vi "UDP Streamer.vi"() -> ()   [LabVIEW 2017]
panel:
  out "#Clients":u32
  in  "Stop":bool
  in  "Delay":i32(knob)=19 caption="Send Packet Every (ms)" min=1 scale=1.0..200.0
  in  "Size":i32(knob)=17515 caption="UDP Data Packet Size (bytes)" min=1 scale=0.0..100000.0 scale format="%#_6p"
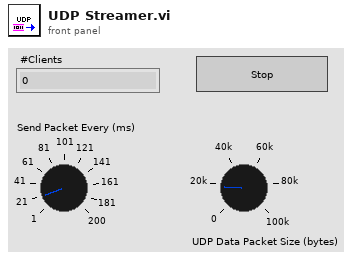
[diagram p1: front panel]
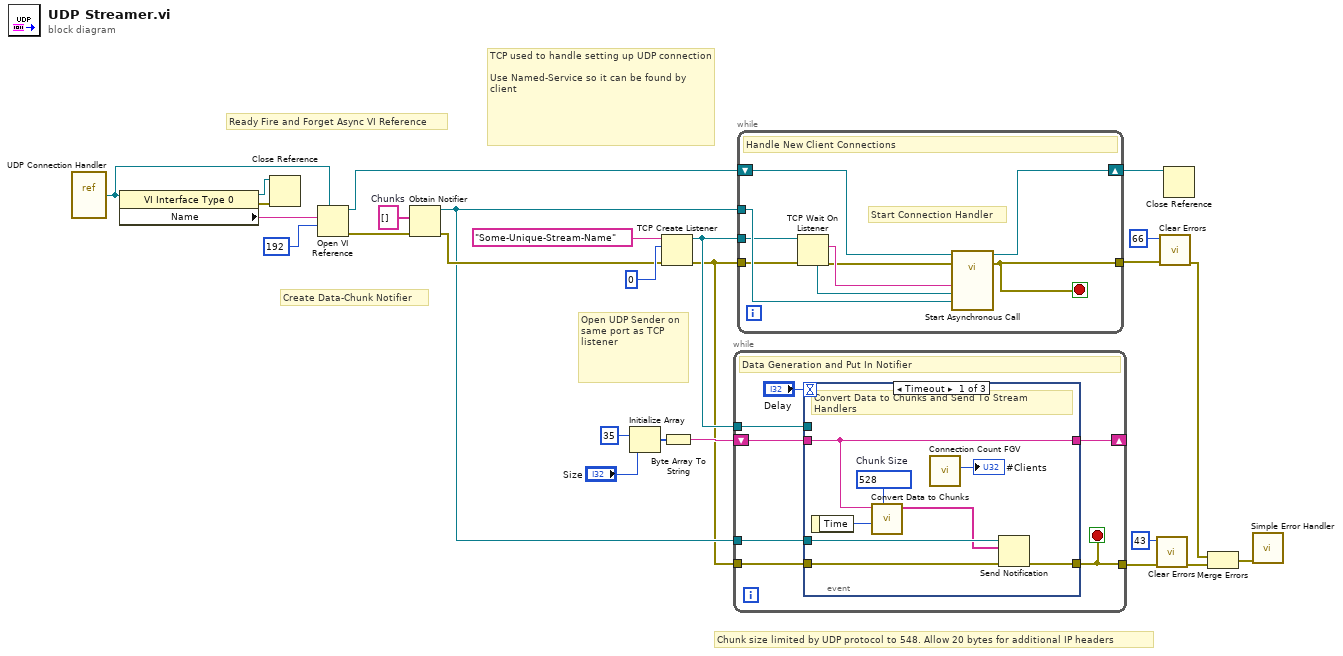
[diagram p0: block diagram]
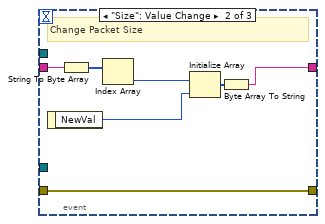
[diagram p2: hidden frame]
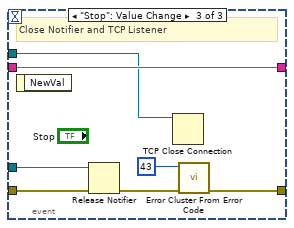
[diagram p3: hidden frame]
diagram:
  w14 = string[] []  # Chunks
  # "Chunk size limited by UDP protocol to 548. Allow 20 bytes for additional IP headers"
  # "Open UDP Sender on same port as TCP listener"
  # "TCP used to handle setting up UDP connection\n\nUse Named-Service so it can be found by client"
  # "Create Data-Chunk Notifier"
  # "Ready Fire and Forget Async VI Reference"
  n1 = vi-ref "UDP Connection Handler.vi"() -> (w10:refnum<vi>)
  n2 = property class="VI Interface Type 0"(reference=w10) -> (reference out=w8:refnum<vi>, error out=w9:errorcluster, "Name"=w11:string)  [unwired: 1 in]
  n3 = Close Reference(reference=w8, error in (no error)=w9) -> ()  [unwired: 1 out]
  n4 = Open VI Reference(type specifier VI Refnum (for type only)=w10, vi path=w11, options=192) -> (vi reference=w5:refnum<vi>, error out=w6:errorcluster)  [unwired: 3 in]
  n5 = Obtain Notifier(notification data type=w14, error in (no error)=w6) -> (notifier out=w12:refnum<notifier>, error out=w13:errorcluster)  [unwired: 2 in, 1 out]
  n6 = Initialize Array(u8 35, "Size") -> (w23:u8[])
  n7 = TCP Create Listener(8:w13, 10:u16 0 ("port"), 11:"Some-Unique-Stream-Name") -> (0:w1:errorcluster, 3:w3:refnum<k5>)  [unwired: 2 in, 1 out]
  n8 = Byte Array To String(unsigned byte array=w23) -> (string=w22:string)
  n9 = while {
    shift-right: [w31] -> _
    shift-left: w22 -> [w33]
    tunnel: w12 -> [w30]
    tunnel: [w29] -> w21
    tunnel: w1 -> [w28]
    tunnel: w3 -> [w27]
    stop <- w29 stop-if-true
    # "Data Generation and Put In Notifier"
    n10 = event shown="[0] Timeout" {
      selector: _ -> [_ _ _]
      dyn-events: _ -> [_ _ _]
      timeout: "Delay" -> [_ _ _]
      tunnel: w33 -> [w37 w45 w53]
      tunnel: [w37 w46 w53] -> w31
      tunnel: [w38 w42 w54] -> w29
      tunnel: w30 -> [w40 _ w55]
      tunnel: w28 -> [w39 w42 w51]
      tunnel: w27 -> [_ _ w49]
      event Timeout {
        w35 = 528  # Chunk Size
        # "Convert Data to Chunks and Send To Stream Handlers"
        n11 = event-data() -> ("Time"=w41:u32)  [unwired: 1 in]
        n12 = call "Convert Data to Chunks.vi"("Chunk Size"=w35, "Chunk ID"=w41, "Data"=w37) -> ("Chunks"=w36:string[])  [unwired: 8 in]
        n13 = call "Connection Count FGV.vi"() -> ("Count"=→"#Clients":u32)  [unwired: 10 in, 1 out]
        n14 = Send Notification(notification=w36, notifier=w40, error in (no error)=w39) -> (error out=w38:errorcluster)  [unwired: 1 out]
      }
      event "Size": Value Change {
        # "Change Packet Size"
        n15 = event-data() -> ("NewVal"=w48:i32)  [unwired: 1 in]
        n16 = String To Byte Array(string=w45) -> (unsigned byte array=w44:u8[])
        n17 = Index Array(array=w44) -> (element=w43:u8)  [unwired: 1 in]
        n18 = Initialize Array(w43, w48) -> (w47:u8[])
        n19 = Byte Array To String(unsigned byte array=w47) -> (string=w46:string)
      }
      event "Stop": Value Change {
        # "Close Notifier and TCP Listener"
        n20 = event-data() -> ()  [unwired: 1 in, 1 out]
        n21 = Release Notifier(notifier=w55, error in (no error)=w51) -> (error out=w50:errorcluster)  [unwired: 1 in, 2 out]
        n22 = TCP Close Connection(connection ID=w49) -> ()  [unwired: 2 in, 2 out]
        n23 = call <vilib>:"Error Cluster From Error Code.vi"("error in (no error)"=w50, "error code (0)"=43) -> ("error out"=w54:errorcluster)  [unwired: 7 in]
      }
    }
  }
  n24 = while {
    tunnel: [w63] -> w18
    tunnel: w12 -> [w62]
    shift-right: [w60] -> w4
    shift-left: w5 -> [w61]
    tunnel: w1 -> [w59]
    tunnel: w3 -> [w58]
    stop <- w63 stop-if-true
    # "Start Connection Handler"
    # "Handle New Client Connections"
    n25 = TCP Wait On Listener(8:w59, 11:w58) -> (0:w57:errorcluster, 2:w64:string, 4:w56:refnum<k5>)  [unwired: 2 in, 2 out]
    n26 = call-by-ref "Start Asynchronous Call"(reference=w61, error in=w57, "Chunks To Send"=w62, "TCP Connection"=w56, "Remote Address"=w64) -> (reference out=w60:refnum<vi>, error out=w63:errorcluster)  [unwired: 9 in]
  }
  n27 = call <vilib>:"Clear Errors.vi"("error in (no error)"=w21, "specific error code to clear (0: all)"=43) -> ("error out"=w16:errorcluster)  [unwired: 4 in, 1 out]
  n28 = call <vilib>:"Clear Errors.vi"("error in (no error)"=w18, "specific error code to clear (0: all)"=66) -> ("error out"=w17:errorcluster)  [unwired: 4 in, 1 out]
  n29 = Close Reference(reference=w4) -> ()  [unwired: 1 in, 1 out]
  n30 = Merge Errors(w17, w16) -> (w15:errorcluster)
  n31 = call <vilib>:"Simple Error Handler.vi"("error in (no error)"=w15) -> ()  [unwired: 4 in, 5 out]
